vi "dfd_SCL_Handshaking.vi"(10 "reset":bool, 11 "input valid":bool) -> (0 "run?":bool, 1 "ready for input":bool, 2 "load":bool, 3 "output valid":bool, 5 "reset for cu":bool, 7 "idx":i16)   [LabVIEW 2017]
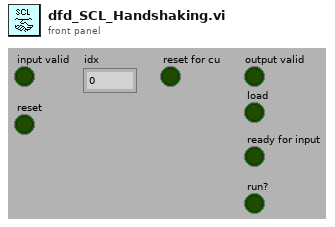
[diagram p1: front panel]
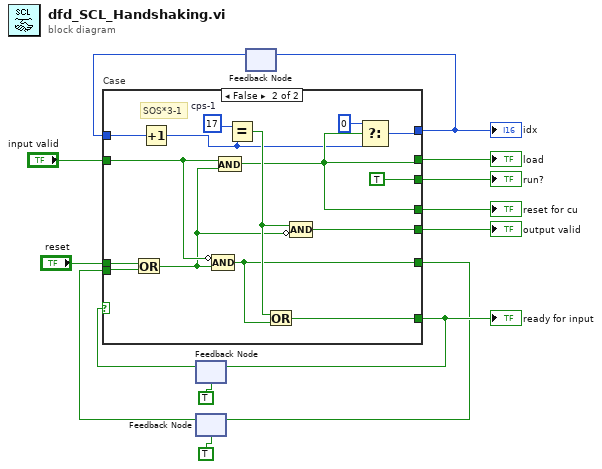
[diagram p0: block diagram]
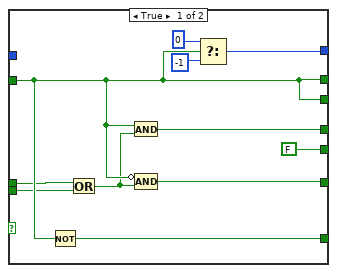
[diagram p2: hidden frame]
diagram:
  n1 = feedback #1(TRUE) -> (w14:bool)
  n2 = feedback #2(TRUE) -> (w1:bool)
  n3 = feedback #3() -> (w7:i16)  [unwired: 1 out]
  n4 = case "Case" shown="False" w14 {
    tunnel: "input valid" -> [w19 w32]
    tunnel: [w19 TRUE ("input valid")] -> w13
    tunnel: [w19 w29] -> w12
    tunnel: [w23 w27] -> w6
    tunnel: w7 -> [_ w39]
    tunnel: [FALSE w37] -> w11
    tunnel: [w21 w36] -> w9
    tunnel: "reset" -> [w16 w33]
    tunnel: [w18 w29] -> w4
    tunnel: [w20 w30] -> w2
    tunnel: w1 -> [w17 w34]
    frame True {
      n5 = Not(x=w19) -> (.not. x?=w21:bool)
      n6 = Or(x=w16, y=w17) -> (x .or. y?=w15:bool)
      n7 = And(x=w19, y=w15) -> (x .and. y?=w18:bool)
      n8 = Compound Arithmetic op=AND(invert w19, w15) -> (w20:bool)
      n9 = Select(t=i16 0, s=w19, f=i16 -1) -> (s? t:f=w23:i16)
    }
    frame False {
      w40 = i16 17  # cps-1
      # "SOS*3-1"
      n10 = Or(x=w33, y=w34) -> (x .or. y?=w31:bool)
      n11 = Increment(x=w39) -> (x+1=w28:i16)
      n12 = Compound Arithmetic op=AND(invert w32, w31) -> (w30:bool)
      n13 = And(x=w32, y=w31) -> (x .and. y?=w29:bool)
      n14 = Equal?(x=w40, y=w28) -> (x = y?=w35:bool)
      n15 = Or(x=w35, y=w30) -> (x .or. y?=w36:bool)
      n16 = Compound Arithmetic op=AND(w35, invert w31) -> (w37:bool)
      n17 = Select(t=i16 0 ("y"), s=w29, f=w28) -> (s? t:f=w27:i16)
    }
  }
  "run?" <- w13
  "ready for input" <- w9
  "load" <- w12
  "output valid" <- w11
  "idx" <- w6
  "reset for cu" <- w4
  n18 = feedback-in #1(w9) -> ()
  n19 = feedback-in #2(w2) -> ()
  n20 = feedback-in #3(w6) -> ()
